vi "Quadrotor PWM.vi"() -> ()   [LabVIEW 2013]
uses:
  <vilib>/Platform/TimedLoop/XDataNode/timing_clust.ctl
  <vilib>/Platform/TimedLoop/XDataNode/nitl_modes.ctl
  <vilib>/Platform/TimedLoop/XDataNode/wakeup.ctl
  <vilib>/FPGAPlugInAG/myRIO-1900/niLvFpga_Open_myRIO-1900.vi
  <vilib>/rvi/interface/common/dynamic/niFpgaDynamicAddResources.vi
  <vilib>/myRIO/Common/Instrument Driver Framework/Utilities/vis/FPGA Ref Manager.vi
  <vilib>/Utility/error.llb/Error Cluster From Error Code.vi
  <vilib>/FPGAPlugInAG/Dynamic/niLvFpga_Close_Dynamic.vi
  <vilib>/rvi/interface/nirviOpenFPGA/nirviOpenFPGA.xnode
  FPGA Bitfiles/MyThirdNImyRIOPr_FPGATarget_myRIO-1900Quadro_Of8fiMD2L+s.lvbitx
  <vilib>/Platform/TimedLoop/XDataNode/XDataNode.xnode
  <vilib>/rvi/interface/nirviCloseFPGA/nirviCloseFPGA.xnode
  <vilib>/myRIO/Instrument Drivers/Utilities/Utilities.lvlib
  <vilib>/Platform/TimedLoop/XDataNode/XDNodeRunTimeDep.lvlib
panel:
  in  "MotorPower":T1 {"PWM3" max=40000 step=5000; "PWM2" max=40000 step=5000; "PWM1" max=40000 step=5000; "PWM0" max=40000 step=5000}
  in  "MotorEN?(F)":bool
  out "error out":errorcluster
  in  "Stop Button":bool
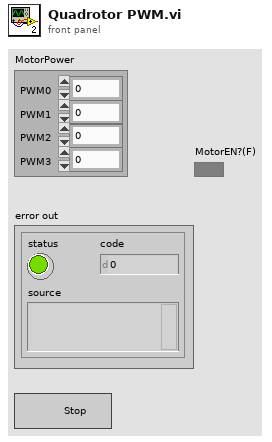
[diagram p1: front panel]
types:
  T1 = cluster{"PWM0":u16, "PWM1":u16, "PWM2":u16, "PWM3":u16}
  T2 = typedef "XDNodeRunTimeDep.lvlib/timing_clust.ctl" = cluster{"Expected End [f-1]":u64, "Actual End [f-1]":u64, "Finished Late? [f-1]":bool, "Expected End [i-1]":u64, "Actual End [i-1]":u64, "Finished Late? [i-1]":bool, "Expected Start [i]":u64, "Actual Start [i]":u64, "Expected Start [f]":u64, "Actual Start [f]":u64, "Source Name":string, "Structure Name":string, "Period":i64, "Deadline":i64, "Offset":i64, "Start":i64, "Priority":i32, "Timeout":i32, "Mode":T3, "Wakeup Reason":T4, "Error":errorcluster, "Source Type":string, "Secondary Source Type":string, "Global End Time":u64, "Global Start Time":u64, "Frame Duration":u64, "Iteration Duration":u64, "Assigned CPU":i32, "I/O Scan Engine Mode":u32}
  T3 = typedef "XDNodeRunTimeDep.lvlib/nitl_modes.ctl" = enum32{"No Change", "Process missed periods, maintain original phase", "Discard missed periods, maintain original phase", "Process missed periods, ignore original phase", "Discard missed periods, ignore original phase"}
  T4 = typedef "XDNodeRunTimeDep.lvlib/wakeup.ctl" = enum32{"Normal", "Aborted", "Asynchronous wakeup", "Timing source error", "Timed loop error", "Timeout"}
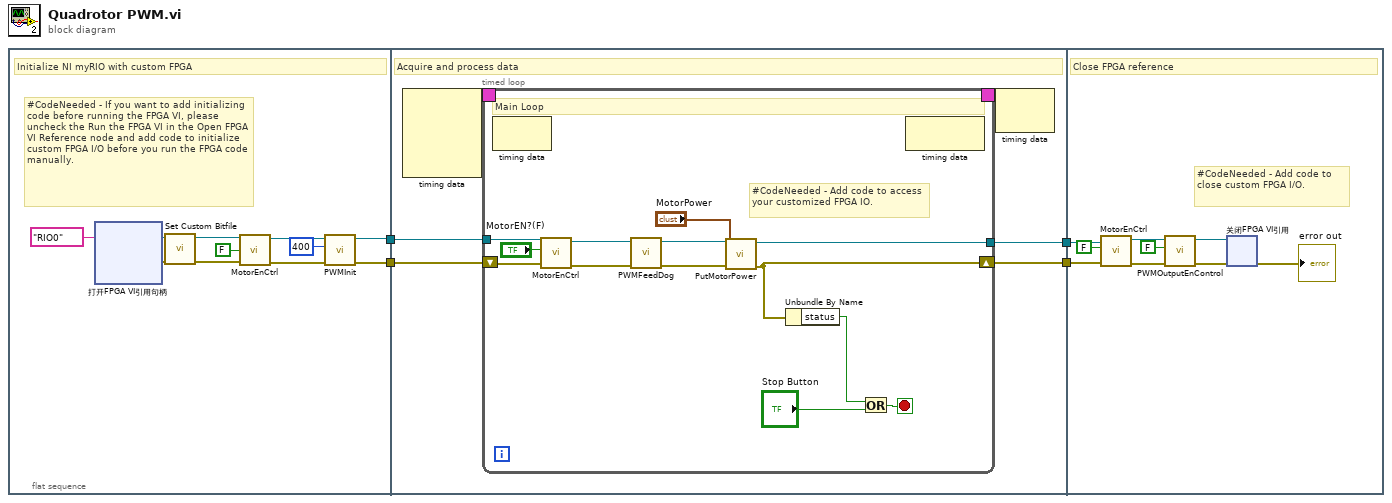
[diagram p0: block diagram]
diagram:
  n1 = flat-sequence {
    tunnel: [w5] -> w4
    tunnel: [w6] -> w2
    tunnel: w4 -> [w21]
    tunnel: [w20] -> w3
    tunnel: w2 -> [w17]
    tunnel: [w16] -> w1
    tunnel: w3 -> [w46]
    tunnel: w1 -> [w43]
    frame #0 {
      # "#CodeNeeded - If you want to add initializing code before running the FPGA VI, please uncheck the Run the FPGA VI in the Open FPGA VI Reference node and add code to initialize custom FPGA I/O before you run the FPGA code manually."
      # "Initialize NI myRIO with custom FPGA"
      n2 = xnode "打开FPGA VI引用句柄"("资源名称"=tag "RIO0" ("resource name")) -> ("FPGA VI引用输出"=w13:refnum<k20>, "错误输出"=w14:errorcluster)  [unwired: 1 in]
      n3 = call <vilib>:"Set Custom Bitfile.vi"("error in (no error)"=w14, "Customized FPGA Reference in"=w13) -> ("error out"=w11:errorcluster, "Customized FPGA Reference out"=w12:refnum<k20>)  [unwired: 8 in]
      n4 = call "MotorEnCtrl.vi"("ErrorIn(no error)"=w11, "MotorEN?(F)"=FALSE, "FPGA VI引用输入"=w12) -> ("ErrorOut"=w9:errorcluster, "FPGA VI引用输出"=w8:refnum<k20>)  [unwired: 7 in]
      n5 = call "PWMInit.vi"("ErrorIn(no error)"=w9, "PMWFreq(200Hz)"=u32 400, "FPGA VI引用输入"=w8) -> ("ErrorOut"=w6:errorcluster, "FPGA VI引用输出"=w5:refnum<k20>)  [unwired: 7 in]
    }
    frame #1 {
      # "Acquire and process data"
      n6 = node-c288() -> (w19:T2)  [unwired: 4 in]
      n7 = timed-loop {
        tunnel: w21 -> [w31]
        shift-right: [w23] -> w20
        shift-left: w17 -> [w30]
        timing: w19 -> [_]
        timing-out: [_] -> w18
        tunnel: [w24] -> w16
        stop <- w33 stop-if-true
        # "#CodeNeeded - Add code to access your customized FPGA IO."
        # "Main Loop"
        n8 = node-c288() -> ()  [unwired: 1 in, 1 out]
        n9 = call "MotorEnCtrl.vi"("ErrorIn(no error)"=w30, "MotorEN?(F)"="MotorEN?(F)", "FPGA VI引用输入"=w31) -> ("ErrorOut"=w29:errorcluster, "FPGA VI引用输出"=w28:refnum<k20>)  [unwired: 7 in]
        n10 = call "PWMFeedDog.vi"("ErrorIn(no error)"=w29, "FPGA VI引用输入"=w28) -> ("ErrorOut"=w27:errorcluster, "FPGA VI引用输出"=w26:refnum<k20>)  [unwired: 8 in]
        n11 = call "PutMotorPower.vi"("ErrorIn(no error)"=w27, "MotorPower"="MotorPower", "FPGA VI引用输入"=w26) -> ("ErrorOut"=w23:errorcluster, "FPGA VI引用输出"=w24:refnum<k20>)  [unwired: 7 in]
        n12 = Unbundle By Name(w23) -> ("status"=w22:bool)
        n13 = Or(x=w22, y="Stop Button") -> (x .or. y?=w33:bool)
        n14 = node-c288() -> ()  [unwired: 1 in, 1 out]
      }
      n15 = node-c288(w18) -> ()  [unwired: 1 out]
    }
    frame #2 {
      # "#CodeNeeded - Add code to close custom FPGA I/O."
      # "Close FPGA reference"
      n16 = call "MotorEnCtrl.vi"("ErrorIn(no error)"=w46, "MotorEN?(F)"=FALSE, "FPGA VI引用输入"=w43) -> ("ErrorOut"=w45:errorcluster, "FPGA VI引用输出"=w42:refnum<k20>)  [unwired: 7 in]
      n17 = call "PWMOutputEnControl.vi"("ErrorIn(no error)"=w45, "OutEN?(F)"=FALSE, "FPGA VI引用输入"=w42) -> ("ErrorOut"=w44:errorcluster, "FPGA VI引用输出"=w41:refnum<k20>)  [unwired: 7 in]
      n18 = xnode "关闭FPGA VI引用"("FPGA VI引用输入"=w41, "错误输入"=w44) -> ("错误输出"=→"error out":errorcluster)
    }
  }
